vi "Init with Value.vi"(8 "error in":errorcluster, 10 "Value":variant, 11 "Image in":refnum<class "Image.lvclass">) -> (0 "error out":errorcluster, 3 "Image out":refnum<class "Image.lvclass">)   [LabVIEW 2024, in "SourceGrid.lvlib" / "Image.lvclass"]
uses:
  Image.lvclass
  D:/git/Sourcegrid-LabVIEW/source/Cells/Cell/Cell.lvclass
  Cell/Cell.lvclass/Cell.ctl
  Image.lvclass/Image.ctl
  Cell/Cell.lvclass
  D:/git/Sourcegrid-LabVIEW/source/Cells/Image/Image.lvclass
  D:/git/Sourcegrid-LabVIEW/dll/SourceGrid.dll
  dll/SourceGrid.dll
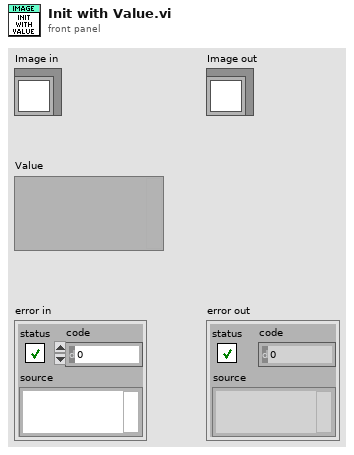
[diagram p1: front panel]
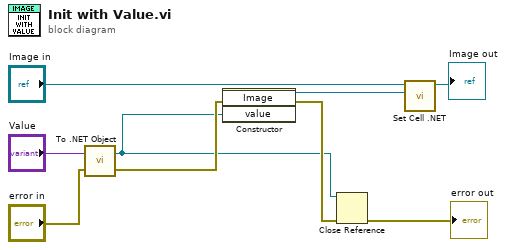
[diagram p0: block diagram]
diagram:
  n1 = call <vilib>:"To .NET Object.vi"("error in (no error)"="error in", "anything"="Value") -> ("error out"=w5:errorcluster, ".NET object"=w2:refnum<k24>)
  n2 = constructor class="Image"(error in=w5, "value"=w2) -> (reference out=w1:refnum<k24>, error out=w9:errorcluster)  [unwired: 2 in, 2 out]
  n3 = Close Reference(reference=w2, error in (no error)=w9) -> (error out=→"error out":errorcluster)
  n4 = call "Set Cell .NET.vi"("Cell .NET"=w1, "Cell in"="Image in") -> ("Cell out"=→"Image out":refnum<class "Image.lvclass">)  [unwired: 9 in]
